vi "Data Logging_Generate Header.vi"(8 "error in":errorcluster, 9 "Include Units\nin Header (F)":bool, 10 "Units of Measure Input":T2, 11 "Data Logging Options":T1={"Absolute Press."=TRUE, "Gauge/Diff. Press."=TRUE, "Barometric Press."=TRUE, "Temperature"=TRUE, "Volumetric"=TRUE, "Mass Flow"=TRUE, "Setpoint"=TRUE, "Valve Drive"=FALSE, "Totalizer"=TRUE, "Tot. Timer [s]"=FALSE, "Tot. Avg. Flow"=FALSE, "Tot. Peak Flow"=FALSE, "Gas Selected"=TRUE, "Log Data"=FALSE}) -> (0 "error out":errorcluster, 3 "Data Log Header":string)   [LabVIEW 2016]
doc: "Generates a header string for use with data logging. Output will be a comma delimited string containing labels of the variables (and the units of measure, if selected) for the data logging options selected."
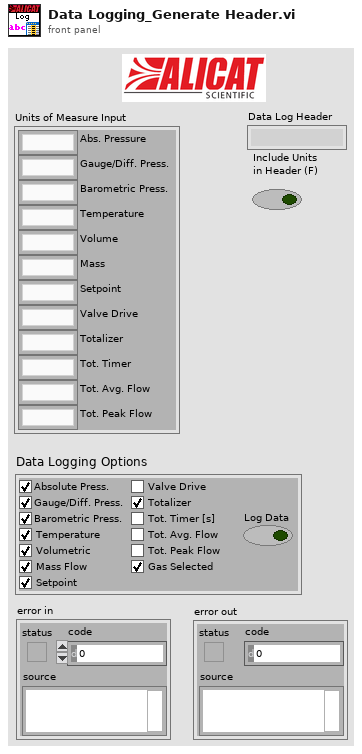
[diagram p1: front panel]
types:
  T1 = cluster{"Absolute Press.":bool, "Gauge/Diff. Press.":bool, "Barometric Press.":bool, "Temperature":bool, "Volumetric":bool, "Mass Flow":bool, "Setpoint":bool, "Valve Drive":bool, "Totalizer":bool, "Tot. Timer [s]":bool, "Tot. Avg. Flow":bool, "Tot. Peak Flow":bool, "Gas Selected":bool, "Log Data":bool}
  T2 = cluster{"Abs. Pressure":string, "Gauge/Diff. Press.":string, "Barometric Press.":string, "Temperature":string, "Volume":string, "Mass":string, "Setpoint":string, "Valve Drive":string, "Totalizer":string, "Tot. Timer":string, "Tot. Avg. Flow":string, "Tot. Peak Flow":string}
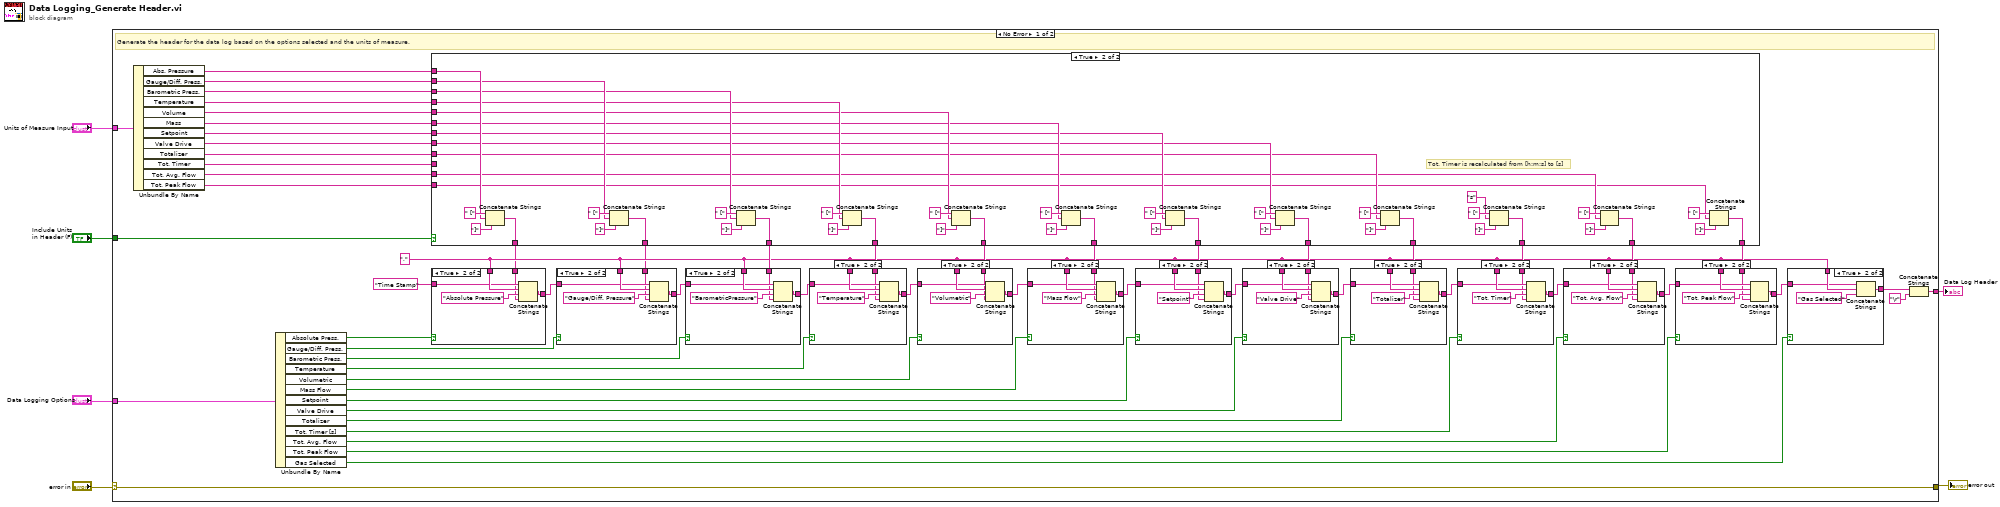
[diagram p0: block diagram]
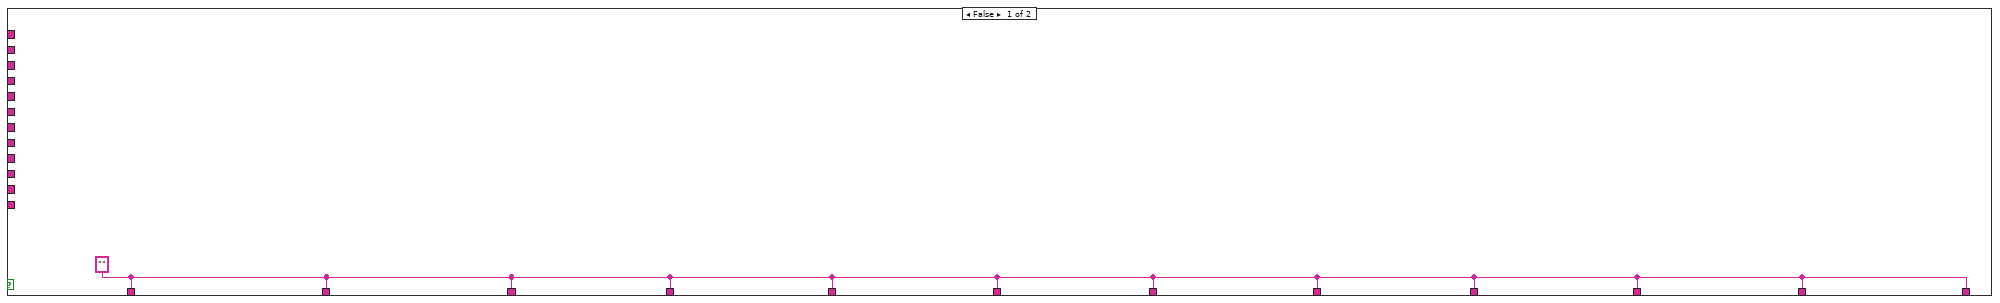
[diagram p4: hidden frame]
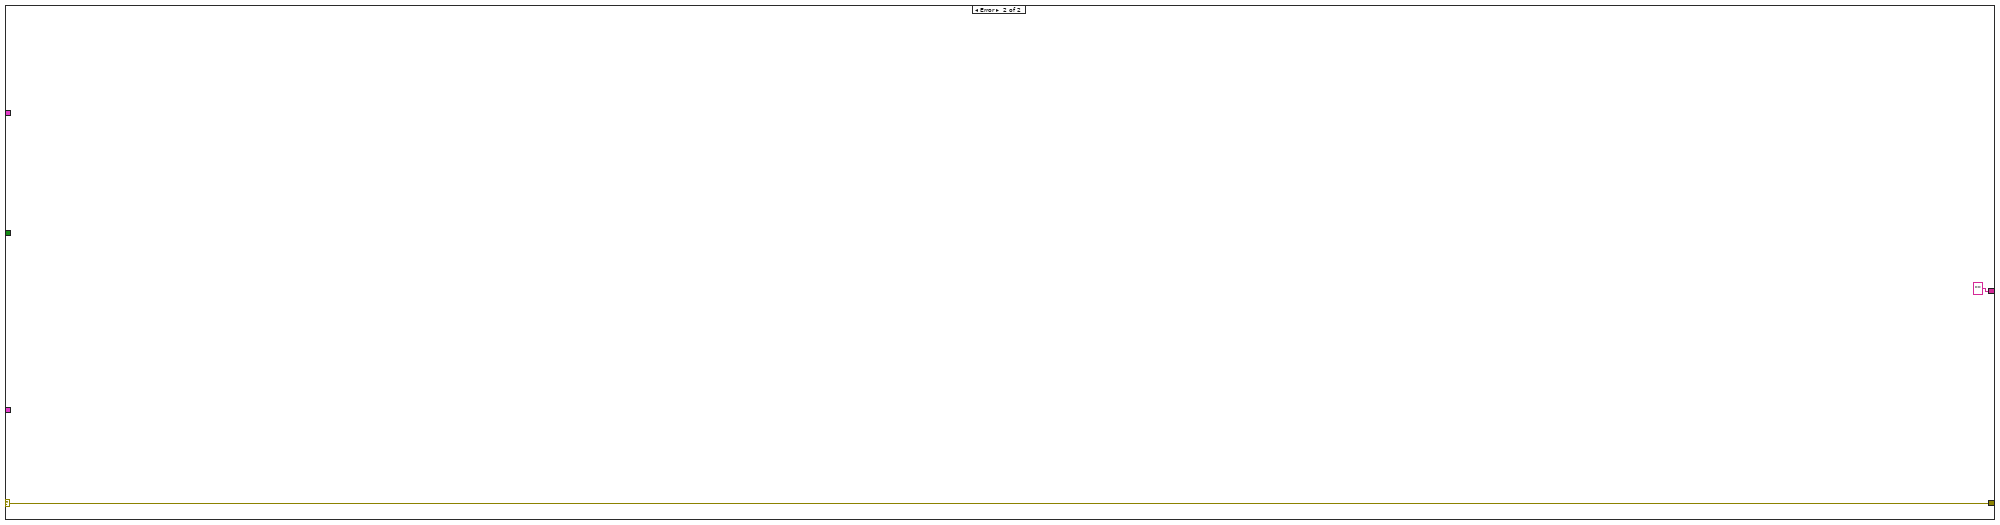
[diagram p16: hidden frame]
diagram:
  n1 = case shown="No Error" "error in" {
    selector: "error in" -> [w43 w191]
    tunnel: "Data Logging Options" -> [w44 _]
    tunnel: [w43 w191] -> w5
    tunnel: "Units of Measure Input" -> [w28 _]
    tunnel: [w41 "" ("string")] -> w4
    tunnel: "Include Units\nin Header (F)" -> [w29 _]
    frame No Error {
      w25 = "," ("string")
      # "Generate the header for the data log based on the options selected and the units of measure."
      n2 = Unbundle By Name(w28) -> ("Abs. Pressure"=w9:string, "Gauge/Diff. Press."=w10:string, "Barometric Press."=w11:string, "Temperature"=w12:string, "Volume"=w13:string, "Mass"=w14:string, "Setpoint"=w15:string, "Valve Drive"=w16:string, "Totalizer"=w17:string, "Tot. Timer"=w18:string, "Tot. Avg. Flow"=w19:string, "Tot. Peak Flow"=w20:string)
      n3 = Unbundle By Name(w44) -> ("Absolute Press."=w23:bool, "Gauge/Diff. Press."=w21:bool, "Barometric Press."=w22:bool, "Temperature"=w54:bool, "Volumetric"=w53:bool, "Mass Flow"=w52:bool, "Setpoint"=w51:bool, "Valve Drive"=w50:bool, "Totalizer"=w49:bool, "Tot. Timer [s]"=w48:bool, "Tot. Avg. Flow"=w47:bool, "Tot. Peak Flow"=w46:bool, "Gas Selected"=w45:bool)
      n4 = case shown="True" w29 {
        tunnel: [w77 w125] -> w39
        tunnel: [w77 w120] -> w38
        tunnel: [w77 w119] -> w37
        tunnel: [w77 w114] -> w35
        tunnel: [w77 w96] -> w36
        tunnel: [w77 w109] -> w34
        tunnel: [w77 w108] -> w33
        tunnel: [w77 w103] -> w32
        tunnel: [w77 w102] -> w31
        tunnel: [w77 w97] -> w30
        tunnel: w20 -> [_ w81]
        tunnel: w19 -> [_ w82]
        tunnel: w18 -> [_ _]
        tunnel: w17 -> [_ w83]
        tunnel: w16 -> [_ w84]
        tunnel: w15 -> [_ w85]
        tunnel: w14 -> [_ w86]
        tunnel: w13 -> [_ w87]
        tunnel: w12 -> [_ w88]
        tunnel: w11 -> [_ w89]
        tunnel: w10 -> [_ w90]
        tunnel: w9 -> [_ w91]
        tunnel: [w77 w79] -> w8
        tunnel: [w77 w78] -> w7
        frame False {
          w77 = ""
          # "no units of measure included"
        }
        frame True {
          # "Tot. Timer is recalculated from [h:m:s] to [s]"
          # "Get the units of measure, if enabled"
          n5 = Concatenate Strings(" [" ("string"), w91, "]" ("string")) -> (w78:string)
          n6 = Concatenate Strings(" [" ("string"), w90, "]" ("string")) -> (w79:string)
          n7 = Concatenate Strings(" [" ("string"), w89, "]" ("string")) -> (w125:string)
          n8 = Concatenate Strings(" [" ("string"), w88, "]" ("string")) -> (w120:string)
          n9 = Concatenate Strings(" [" ("string"), w87, "]" ("string")) -> (w119:string)
          n10 = Concatenate Strings(" [" ("string"), w86, "]" ("string")) -> (w114:string)
          n11 = Concatenate Strings(" [" ("string"), w85, "]" ("string")) -> (w96:string)
          n12 = Concatenate Strings(" [" ("string"), w84, "]" ("string")) -> (w109:string)
          n13 = Concatenate Strings(" [" ("string"), w83, "]" ("string")) -> (w108:string)
          n14 = Concatenate Strings(" [" ("string"), "s" ("string"), "]" ("string")) -> (w103:string)
          n15 = Concatenate Strings(" [" ("string"), w82, "]" ("string")) -> (w102:string)
          n16 = Concatenate Strings(" [" ("string"), w81, "]" ("string")) -> (w97:string)
        }
      }
      n17 = case shown="True" w23 {
        tunnel: "Time Stamp" ("string") -> [w65 w67]
        tunnel: [w65 w70] -> w27
        tunnel: w25 -> [_ w68]
        tunnel: w7 -> [_ w66]
        frame False {
        }
        frame True {
          n18 = Concatenate Strings(w67, w68, "Absolute Pressure" ("string"), w66) -> (w70:string)
        }
      }
      n19 = case shown="True" w21 {
        tunnel: w27 -> [w71 w73]
        tunnel: [w71 w76] -> w26
        tunnel: w25 -> [_ w74]
        tunnel: w8 -> [_ w72]
        frame False {
        }
        frame True {
          n20 = Concatenate Strings(w73, w74, "Gauge/Diff. Pressure" ("string"), w72) -> (w76:string)
        }
      }
      n21 = case shown="True" w22 {
        tunnel: w26 -> [w185 w187]
        tunnel: [w185 w190] -> w64
        tunnel: w25 -> [_ w188]
        tunnel: w39 -> [_ w186]
        frame False {
        }
        frame True {
          n22 = Concatenate Strings(w187, w188, "BarometricPressure" ("string"), w186) -> (w190:string)
        }
      }
      n23 = case shown="True" w54 {
        tunnel: w64 -> [w179 w181]
        tunnel: [w179 w184] -> w56
        tunnel: w25 -> [_ w182]
        tunnel: w38 -> [_ w180]
        frame False {
        }
        frame True {
          n24 = Concatenate Strings(w181, w182, "Temperature" ("string"), w180) -> (w184:string)
        }
      }
      n25 = case shown="True" w53 {
        tunnel: w56 -> [w173 w175]
        tunnel: [w173 w178] -> w55
        tunnel: w25 -> [_ w176]
        tunnel: w37 -> [_ w174]
        frame False {
        }
        frame True {
          n26 = Concatenate Strings(w175, w176, "Volumetric" ("string"), w174) -> (w178:string)
        }
      }
      n27 = case shown="True" w52 {
        tunnel: w55 -> [w167 w169]
        tunnel: [w167 w172] -> w63
        tunnel: w25 -> [_ w170]
        tunnel: w35 -> [_ w168]
        frame False {
        }
        frame True {
          n28 = Concatenate Strings(w169, w170, "Mass Flow" ("string"), w168) -> (w172:string)
        }
      }
      n29 = case shown="True" w51 {
        tunnel: w63 -> [w161 w163]
        tunnel: [w161 w166] -> w62
        tunnel: w25 -> [_ w164]
        tunnel: w36 -> [_ w162]
        frame False {
        }
        frame True {
          n30 = Concatenate Strings(w163, w164, "Setpoint" ("string"), w162) -> (w166:string)
        }
      }
      n31 = case shown="True" w50 {
        tunnel: w62 -> [w155 w157]
        tunnel: [w155 w160] -> w61
        tunnel: w25 -> [_ w158]
        tunnel: w34 -> [_ w156]
        frame False {
        }
        frame True {
          n32 = Concatenate Strings(w157, w158, "Valve Drive" ("string"), w156) -> (w160:string)
        }
      }
      n33 = case shown="True" w49 {
        tunnel: w61 -> [w149 w151]
        tunnel: [w149 w154] -> w60
        tunnel: w25 -> [_ w152]
        tunnel: w33 -> [_ w150]
        frame False {
        }
        frame True {
          n34 = Concatenate Strings(w151, w152, "Totalizer" ("string"), w150) -> (w154:string)
        }
      }
      n35 = case shown="True" w48 {
        tunnel: w60 -> [w143 w145]
        tunnel: [w143 w148] -> w59
        tunnel: w25 -> [_ w146]
        tunnel: w32 -> [_ w144]
        frame False {
        }
        frame True {
          n36 = Concatenate Strings(w145, w146, "Tot. Timer" ("string"), w144) -> (w148:string)
        }
      }
      n37 = case shown="True" w47 {
        tunnel: w59 -> [w137 w139]
        tunnel: [w137 w142] -> w58
        tunnel: w25 -> [_ w140]
        tunnel: w31 -> [_ w138]
        frame False {
        }
        frame True {
          n38 = Concatenate Strings(w139, w140, "Tot. Avg. Flow" ("string"), w138) -> (w142:string)
        }
      }
      n39 = case shown="True" w46 {
        tunnel: w58 -> [w131 w133]
        tunnel: [w131 w136] -> w57
        tunnel: w25 -> [_ w134]
        tunnel: w30 -> [_ w132]
        frame False {
        }
        frame True {
          n40 = Concatenate Strings(w133, w134, "Tot. Peak Flow" ("string"), w132) -> (w136:string)
        }
      }
      n41 = case shown="True" w45 {
        tunnel: w57 -> [w126 w127]
        tunnel: [w126 w130] -> w42
        tunnel: w25 -> [_ w128]
        frame False {
        }
        frame True {
          n42 = Concatenate Strings(w127, w128, "Gas Selected" ("string")) -> (w130:string)
        }
      }
      n43 = Concatenate Strings(w42, "\r" ("string")) -> (w41:string)
    }
    frame Error {
    }
  }
  "error out" <- w5
  "Data Log Header" <- w4
